vi "Write Test Configuration (INI) File_MultiTest.vi"(1 "# of Cycles(No \"T\")":string, 5 "ListBox_Selected_Tests":T1, 7 "FilePath in":path=path "C:/Users/DalLab/Desktop/Test Data", 10 "Filename: Date_LOT_Design_\"RCV\"":string, 11 "Experiments":T2={"Exp 1"={"Floor_Sweep_Stop_V"=36.0, "Resistance Threshold"=1000.0, "Floor_Sweep_Start_V"=0.0, "Floor_Sweep_Step_V"=1.0, "Roof_Sweep_Stop_V"=36.0, "Roof_Sweep_Start_V"=0.0, "Roof_Sweep_Step_V"=1.0, "Experiment Name"="", "Meas_Type"=[0, 2, 4]}, "Exp 2"={"Floor_Sweep_Stop_V"=36.0, "Resistance Threshold"=1000.0, "Floor_Sweep_Start_V"=0.0, "Floor_Sweep_Step_V"=1.0, "Roof_Sweep_Stop_V"=36.0, "Roof_Sweep_Start_V"=0.0, "Roof_Sweep_Step_V"=1.0, "Experiment Name"="", "Meas_Type"=[0, 2, 4]}, "Exp 3"={"Floor_Sweep_Stop_V"=36.0, "Resistance Threshold"=1000.0, "Floor_Sweep_Start_V"=0.0, "Floor_Sweep_Step_V"=1.0, "Roof_Sweep_Stop_V"=36.0, "Roof_Sweep_Start_V"=0.0, "Roof_Sweep_Step_V"=1.0, "Experiment Name"="", "Meas_Type"=[0, 2, 4]}, "Exp 4"={"Floor_Sweep_Stop_V"=36.0, "Resistance Threshold"=1000.0, "Floor_Sweep_Start_V"=0.0, "Floor_Sweep_Step_V"=1.0, "Roof_Sweep_Stop_V"=36.0, "Roof_Sweep_Start_V"=0.0, "Roof_Sweep_Step_V"=1.0, "Experiment Name"="", "Meas_Type"=[0, 2, 4]}}) -> (2 "Hold Down Time(Seconds) 2":dbl, 3 "Final Filepath Out":path)   [LabVIEW 2013]
doc: "Setup up to 4 different experiments. During SDR setup the specific experiments will be selected."
uses:
  Support/Controls/Multiple Exp Setup_MultiTest.ctl
  Support/Controls/Individual User Inputs_MultiTest.ctl
  Support/Controls/Test Selection.ctl
  <vilib>/Utility/config.llb/Write Key (String).vi
  <vilib>/Utility/config.llb/Write Key (Double).vi
  <vilib>/Utility/config.llb/Write Key (Path).vi
  <vilib>/Utility/config.llb/NI_LVConfig.lvlib
panel:
  in  "Hold Down Time(Seconds)":dbl=15.0
  in  "Save Button":bool
  # "Calculation Settings"
  # "Test Settings"
  # "Calculation Settings"
  # "Test Settings"
  # "Calculation Settings"
  # "Test Settings"
  # "Calculation Settings"
  # "Test Settings"
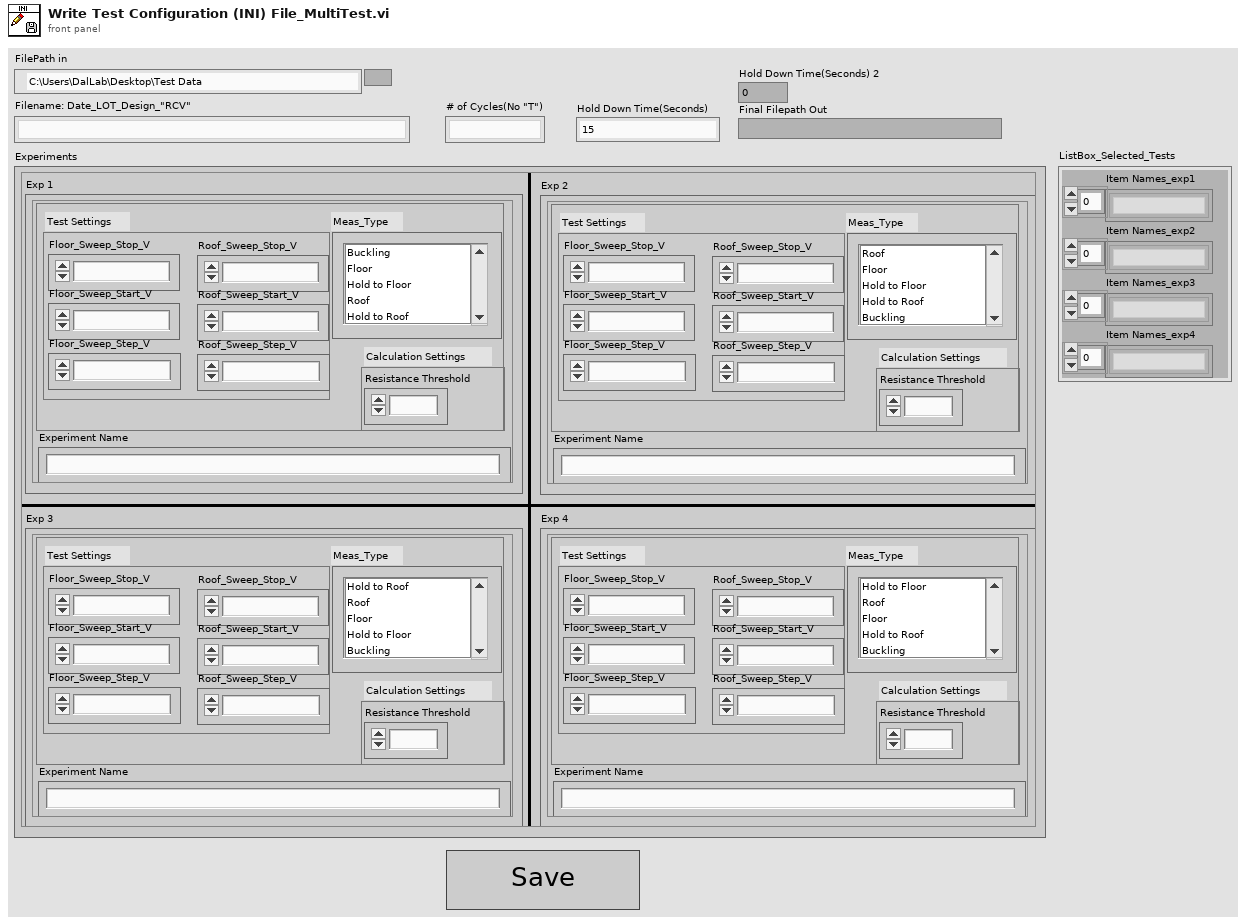
[diagram p1: front panel]
types:
  T1 = cluster{"Item Names_exp1":string[], "Item Names_exp2":string[], "Item Names_exp3":string[], "Item Names_exp4":string[]}
  T2 = typedef "Multiple Exp Setup_MultiTest.ctl" = cluster{"Exp 1":T3, "Exp 2":T3, "Exp 3":T3, "Exp 4":T3}
  T3 = typedef "Individual User Inputs_MultiTest.ctl" = cluster{"Floor_Sweep_Stop_V":dbl, "Resistance Threshold":dbl, "Floor_Sweep_Start_V":dbl, "Floor_Sweep_Step_V":dbl, "Roof_Sweep_Stop_V":dbl, "Roof_Sweep_Start_V":dbl, "Roof_Sweep_Step_V":dbl, "Experiment Name":string, "Meas_Type":T4}
  T4 = typedef "Test Selection.ctl" = i32[]
  T5 = typedef "NI_LVConfig.lvlib/Config Data RefNum.ctl" = refnum<k1>
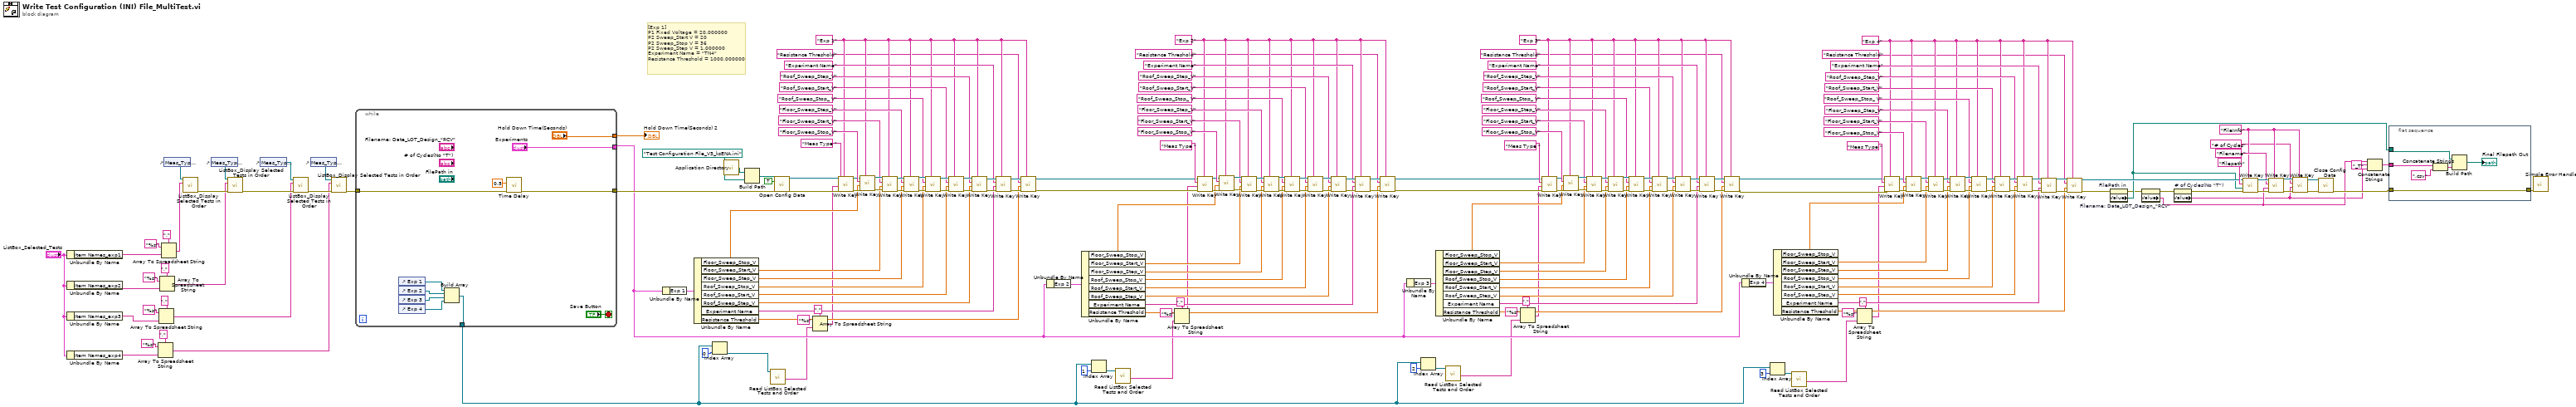
[diagram p0: block diagram]
diagram:
  w49 = "FileInfo" ("section")
  w114 = "Exp 4" ("section")
  w140 = "Exp 3" ("section")
  w166 = "Exp 2" ("section")
  w191 = "Exp 1" ("section")
  # "[Exp 1]\nP1 Fixed Voltage = 20.000000\nP2 Sweep_Start V = 20 \nP2 Sweep_Stop V = 36   \nP2 Sweep_Step V = 1.000000    \nExperiment Name = \"TN4\"\nResistance Threshold = 1000.000000"
  n1 = Unbundle By Name("ListBox_Selected_Tests") -> ("Item Names_exp1"=w22:string[])
  n2 = Unbundle By Name("ListBox_Selected_Tests") -> ("Item Names_exp2"=w9:string[])
  n3 = Unbundle By Name("ListBox_Selected_Tests") -> ("Item Names_exp3"=w6:string[])
  n4 = Unbundle By Name("ListBox_Selected_Tests") -> ("Item Names_exp4"=w7:string[])
  n5 = Array To Spreadsheet String(delimiter (Tab)=",", array=w7, 3:"%s" ("format string")) -> (spreadsheet string=w1:string)
  n6 = Array To Spreadsheet String(delimiter (Tab)=",", array=w6, 3:"%s" ("format string")) -> (spreadsheet string=w4:string)
  n7 = Array To Spreadsheet String(delimiter (Tab)=",", array=w9, 3:"%s" ("format string")) -> (spreadsheet string=w5:string)
  n8 = Array To Spreadsheet String(delimiter (Tab)=",", array=w22, 3:"%s" ("format string")) -> (spreadsheet string=w17:string)
  n9 = control-ref of="Meas_Type_Exp1"() -> (w18:refnum<vi>)
  n10 = call "ListBox_Display Selected Tests in Order.vi"("Tests"=w17, "Meas_Type_exp1"=w18) -> ("Error Out"=w19:errorcluster)  [unwired: 7 in, 2 out]
  n11 = control-ref of="Meas_Type_Exp2"() -> (w16:refnum<vi>)
  n12 = call "ListBox_Display Selected Tests in Order.vi"("Error In"=w19, "Tests"=w5, "Meas_Type_exp1"=w16) -> ("Error Out"=w20:errorcluster)  [unwired: 6 in, 2 out]
  n13 = control-ref of="Meas_Type_Exp3"() -> (w3:refnum<vi>)
  n14 = call "ListBox_Display Selected Tests in Order.vi"("Error In"=w20, "Tests"=w4, "Meas_Type_exp1"=w3) -> ("Error Out"=w21:errorcluster)  [unwired: 6 in, 2 out]
  n15 = control-ref of="Meas_Type_Exp4"() -> (w2:refnum<vi>)
  n16 = call "ListBox_Display Selected Tests in Order.vi"("Error In"=w21, "Tests"=w1, "Meas_Type_exp1"=w2) -> ("Error Out"=w25:errorcluster)  [unwired: 6 in, 2 out]
  n17 = while {
    tunnel: [w238] -> w219
    tunnel: ["Experiments"] -> w110
    tunnel: ["Hold Down Time(Seconds)"] -> w54
    tunnel: [w229] -> w37
    tunnel: w25 -> [w228]
    stop <- "Save Button" stop-if-true
    n18 = control-ref of="Exp 1"() -> (w233:refnum<vi>)
    n19 = control-ref of="Exp 2"() -> (w232:refnum<vi>)
    n20 = control-ref of="Exp 3"() -> (w231:refnum<vi>)
    n21 = control-ref of="Exp 4"() -> (w230:refnum<vi>)
    n22 = Build Array(w233, w232, w231, w230) -> (w229:refnum<vi>[])
    n23 = call "Time Delay"("error in (no error)"=w228, "Delay Time (s)"=0.5) -> ("error out"=w238:errorcluster)  [unwired: 9 in]
  }
  "Hold Down Time(Seconds) 2" <- w54
  n24 = Unbundle By Name(w110) -> ("Exp 1"=w210:T3)
  n25 = Unbundle By Name(w210) -> ("Floor_Sweep_Stop_V"=w208:dbl, "Floor_Sweep_Start_V"=w206:dbl, "Floor_Sweep_Step_V"=w204:dbl, "Roof_Sweep_Stop_V"=w202:dbl, "Roof_Sweep_Start_V"=w200:dbl, "Roof_Sweep_Step_V"=w198:dbl, "Experiment Name"=w192:string, "Resistance Threshold"=w189:dbl)
  n26 = Index Array(array=w37, index=0) -> (element=w26:refnum<vi>)
  n27 = call <vilib>:"Application Directory.vi"() -> ("Application Directory"=w222:path)
  n28 = Build Path(base path=w222, name or relative path=path "Test Configuration File_V3_ksENA.ini" ("default name")) -> (appended path=w223:path)
  n29 = call "Read ListBox Selected Tests and Order.vi"("Experiment Cluster"=w26) -> ("Per Exp Tests to Run"=w47:string[])  [unwired: 7 in, 3 out]
  n30 = call <vilib>:"Open Config Data.vi"("error in (no error)"=w219, "create file if necessary (T)"=TRUE ("create file if necessary? (T)"), "configuration file path"=w223) -> ("error out"=w70:errorcluster, "refnum"=w84:T5)  [unwired: 6 in, 1 out]
  n31 = Array To Spreadsheet String(delimiter (Tab)=",", array=w47, 3:"%s" ("format string")) -> (spreadsheet string=w69:string)
  n32 = call-poly <vilib>:"Write Key.vi"("section"=w191, "error in (no error)"=w70, "value"=w69, "key"="Meas Type " ("Key 1"), "refnum"=w84) -> ("error out"=w212:errorcluster, "refnum out"=w83:T5)  [unwired: 4 in, 1 out]
  n33 = call-poly <vilib>:"Write Key.vi"("section"=w191, "error in (no error)"=w212, "value"=w208, "key"="Floor_Sweep_Stop_V" ("Key 2"), "refnum"=w83) -> ("error out"=w218:errorcluster, "refnum out"=w217:T5)  [unwired: 4 in, 1 out]
  n34 = call-poly <vilib>:"Write Key.vi"("section"=w191, "error in (no error)"=w218, "value"=w206, "key"="Floor_Sweep_Start_V" ("Key 2"), "refnum"=w217) -> ("error out"=w215:errorcluster, "refnum out"=w216:T5)  [unwired: 4 in, 1 out]
  n35 = call-poly <vilib>:"Write Key.vi"("section"=w191, "error in (no error)"=w215, "value"=w204, "key"="Floor_Sweep_Step_V" ("Key 2"), "refnum"=w216) -> ("error out"=w224:errorcluster, "refnum out"=w225:T5)  [unwired: 4 in, 1 out]
  n36 = call-poly <vilib>:"Write Key.vi"("section"=w191, "error in (no error)"=w224, "value"=w202, "key"="Roof_Sweep_Stop_ V" ("Key 3"), "refnum"=w225) -> ("error out"=w221:errorcluster, "refnum out"=w220:T5)  [unwired: 4 in, 1 out]
  n37 = call-poly <vilib>:"Write Key.vi"("section"=w191, "error in (no error)"=w221, "value"=w200, "key"="Roof_Sweep_Start_V" ("Key 3"), "refnum"=w220) -> ("error out"=w214:errorcluster, "refnum out"=w213:T5)  [unwired: 4 in, 1 out]
  n38 = call-poly <vilib>:"Write Key.vi"("section"=w191, "error in (no error)"=w214, "value"=w198, "key"="Roof_Sweep_Step_V" ("Key 3"), "refnum"=w213) -> ("error out"=w196:errorcluster, "refnum out"=w195:T5)  [unwired: 4 in, 1 out]
  n39 = call-poly <vilib>:"Write Key.vi"("section"=w191, "error in (no error)"=w196, "value"=w192, "key"="Experiment Name" ("Key 3"), "refnum"=w195) -> ("error out"=w197:errorcluster, "refnum out"=w194:T5)  [unwired: 4 in, 1 out]
  n40 = call-poly <vilib>:"Write Key.vi"("section"=w191, "error in (no error)"=w197, "value"=w189, "key"="Resistance Threshold" ("Key 3"), "refnum"=w194) -> ("error out"=w63:errorcluster, "refnum out"=w82:T5)  [unwired: 4 in, 1 out]
  n41 = Unbundle By Name(w110) -> ("Exp 2"=w164:T3)
  n42 = Unbundle By Name(w164) -> ("Floor_Sweep_Stop_V"=w109:dbl, "Floor_Sweep_Start_V"=w108:dbl, "Floor_Sweep_Step_V"=w107:dbl, "Roof_Sweep_Stop_V"=w106:dbl, "Roof_Sweep_Start_V"=w105:dbl, "Roof_Sweep_Step_V"=w104:dbl, "Experiment Name"=w103:string, "Resistance Threshold"=w102:dbl)
  n43 = Index Array(array=w37, index=1) -> (element=w41:refnum<vi>)
  n44 = call "Read ListBox Selected Tests and Order.vi"("Experiment Cluster"=w41) -> ("Per Exp Tests to Run"=w46:string[])  [unwired: 7 in, 3 out]
  n45 = Array To Spreadsheet String(delimiter (Tab)=",", array=w46, 3:"%s" ("format string")) -> (spreadsheet string=w61:string)
  n46 = call-poly <vilib>:"Write Key.vi"("section"=w166, "error in (no error)"=w63, "value"=w61, "key"="Meas Type " ("Key 1"), "refnum"=w82) -> ("error out"=w178:errorcluster, "refnum out"=w81:T5)  [unwired: 4 in, 1 out]
  n47 = call-poly <vilib>:"Write Key.vi"("section"=w166, "error in (no error)"=w178, "value"=w109, "key"="Floor_Sweep_Stop_V" ("Key 2"), "refnum"=w81) -> ("error out"=w184:errorcluster, "refnum out"=w183:T5)  [unwired: 4 in, 1 out]
  n48 = call-poly <vilib>:"Write Key.vi"("section"=w166, "error in (no error)"=w184, "value"=w108, "key"="Floor_Sweep_Start_V" ("Key 2"), "refnum"=w183) -> ("error out"=w181:errorcluster, "refnum out"=w182:T5)  [unwired: 4 in, 1 out]
  n49 = call-poly <vilib>:"Write Key.vi"("section"=w166, "error in (no error)"=w181, "value"=w107, "key"="Floor_Sweep_Step_V" ("Key 2"), "refnum"=w182) -> ("error out"=w187:errorcluster, "refnum out"=w188:T5)  [unwired: 4 in, 1 out]
  n50 = call-poly <vilib>:"Write Key.vi"("section"=w166, "error in (no error)"=w187, "value"=w106, "key"="Roof_Sweep_Stop_ V" ("Key 3"), "refnum"=w188) -> ("error out"=w186:errorcluster, "refnum out"=w185:T5)  [unwired: 4 in, 1 out]
  n51 = call-poly <vilib>:"Write Key.vi"("section"=w166, "error in (no error)"=w186, "value"=w105, "key"="Roof_Sweep_Start_V" ("Key 3"), "refnum"=w185) -> ("error out"=w180:errorcluster, "refnum out"=w179:T5)  [unwired: 4 in, 1 out]
  n52 = call-poly <vilib>:"Write Key.vi"("section"=w166, "error in (no error)"=w180, "value"=w104, "key"="Roof_Sweep_Step_V" ("Key 3"), "refnum"=w179) -> ("error out"=w170:errorcluster, "refnum out"=w169:T5)  [unwired: 4 in, 1 out]
  n53 = call-poly <vilib>:"Write Key.vi"("section"=w166, "error in (no error)"=w170, "value"=w103, "key"="Experiment Name" ("Key 3"), "refnum"=w169) -> ("error out"=w171:errorcluster, "refnum out"=w168:T5)  [unwired: 4 in, 1 out]
  n54 = call-poly <vilib>:"Write Key.vi"("section"=w166, "error in (no error)"=w171, "value"=w102, "key"="Resistance Threshold" ("Key 3"), "refnum"=w168) -> ("error out"=w60:errorcluster, "refnum out"=w80:T5)  [unwired: 4 in, 1 out]
  n55 = Unbundle By Name(w110) -> ("Exp 3"=w137:T3)
  n56 = Index Array(array=w37, index=2) -> (element=w39:refnum<vi>)
  n57 = Unbundle By Name(w137) -> ("Floor_Sweep_Stop_V"=w101:dbl, "Floor_Sweep_Start_V"=w100:dbl, "Floor_Sweep_Step_V"=w99:dbl, "Roof_Sweep_Stop_V"=w98:dbl, "Roof_Sweep_Start_V"=w97:dbl, "Roof_Sweep_Step_V"=w96:dbl, "Experiment Name"=w95:string, "Resistance Threshold"=w94:dbl)
  n58 = call "Read ListBox Selected Tests and Order.vi"("Experiment Cluster"=w39) -> ("Per Exp Tests to Run"=w45:string[])  [unwired: 7 in, 3 out]
  n59 = Array To Spreadsheet String(delimiter (Tab)=",", array=w45, 3:"%s" ("format string")) -> (spreadsheet string=w58:string)
  n60 = call-poly <vilib>:"Write Key.vi"("section"=w140, "error in (no error)"=w60, "value"=w58, "key"="Meas Type " ("Key 1"), "refnum"=w80) -> ("error out"=w152:errorcluster, "refnum out"=w85:T5)  [unwired: 4 in, 1 out]
  n61 = call-poly <vilib>:"Write Key.vi"("section"=w140, "error in (no error)"=w152, "value"=w101, "key"="Floor_Sweep_Stop_V" ("Key 2"), "refnum"=w85) -> ("error out"=w158:errorcluster, "refnum out"=w157:T5)  [unwired: 4 in, 1 out]
  n62 = call-poly <vilib>:"Write Key.vi"("section"=w140, "error in (no error)"=w158, "value"=w100, "key"="Floor_Sweep_Start_V" ("Key 2"), "refnum"=w157) -> ("error out"=w155:errorcluster, "refnum out"=w156:T5)  [unwired: 4 in, 1 out]
  n63 = call-poly <vilib>:"Write Key.vi"("section"=w140, "error in (no error)"=w155, "value"=w99, "key"="Floor_Sweep_Step_V" ("Key 2"), "refnum"=w156) -> ("error out"=w161:errorcluster, "refnum out"=w162:T5)  [unwired: 4 in, 1 out]
  n64 = call-poly <vilib>:"Write Key.vi"("section"=w140, "error in (no error)"=w161, "value"=w98, "key"="Roof_Sweep_Stop_ V" ("Key 3"), "refnum"=w162) -> ("error out"=w160:errorcluster, "refnum out"=w159:T5)  [unwired: 4 in, 1 out]
  n65 = call-poly <vilib>:"Write Key.vi"("section"=w140, "error in (no error)"=w160, "value"=w97, "key"="Roof_Sweep_Start_V" ("Key 3"), "refnum"=w159) -> ("error out"=w154:errorcluster, "refnum out"=w153:T5)  [unwired: 4 in, 1 out]
  n66 = call-poly <vilib>:"Write Key.vi"("section"=w140, "error in (no error)"=w154, "value"=w96, "key"="Roof_Sweep_Step_V" ("Key 3"), "refnum"=w153) -> ("error out"=w144:errorcluster, "refnum out"=w143:T5)  [unwired: 4 in, 1 out]
  n67 = call-poly <vilib>:"Write Key.vi"("section"=w140, "error in (no error)"=w144, "value"=w95, "key"="Experiment Name" ("Key 3"), "refnum"=w143) -> ("error out"=w145:errorcluster, "refnum out"=w142:T5)  [unwired: 4 in, 1 out]
  n68 = call-poly <vilib>:"Write Key.vi"("section"=w140, "error in (no error)"=w145, "value"=w94, "key"="Resistance Threshold" ("Key 3"), "refnum"=w142) -> ("error out"=w57:errorcluster, "refnum out"=w79:T5)  [unwired: 4 in, 1 out]
  n69 = Unbundle By Name(w110) -> ("Exp 4"=w111:T3)
  n70 = Index Array(array=w37, index=3) -> (element=w36:refnum<vi>)
  n71 = Unbundle By Name(w111) -> ("Floor_Sweep_Stop_V"=w93:dbl, "Floor_Sweep_Start_V"=w92:dbl, "Floor_Sweep_Step_V"=w91:dbl, "Roof_Sweep_Stop_V"=w90:dbl, "Roof_Sweep_Start_V"=w89:dbl, "Roof_Sweep_Step_V"=w88:dbl, "Experiment Name"=w87:string, "Resistance Threshold"=w86:dbl)
  n72 = call "Read ListBox Selected Tests and Order.vi"("Experiment Cluster"=w36) -> ("Per Exp Tests to Run"=w44:string[])  [unwired: 7 in, 3 out]
  n73 = Array To Spreadsheet String(delimiter (Tab)=",", array=w44, 3:"%s" ("format string")) -> (spreadsheet string=w55:string)
  n74 = call-poly <vilib>:"Write Key.vi"("section"=w114, "error in (no error)"=w57, "value"=w55, "key"="Meas Type " ("Key 1"), "refnum"=w79) -> ("error out"=w126:errorcluster, "refnum out"=w78:T5)  [unwired: 4 in, 1 out]
  n75 = call-poly <vilib>:"Write Key.vi"("section"=w114, "error in (no error)"=w126, "value"=w93, "key"="Floor_Sweep_Stop_V" ("Key 2"), "refnum"=w78) -> ("error out"=w132:errorcluster, "refnum out"=w131:T5)  [unwired: 4 in, 1 out]
  n76 = call-poly <vilib>:"Write Key.vi"("section"=w114, "error in (no error)"=w132, "value"=w92, "key"="Floor_Sweep_Start_V" ("Key 2"), "refnum"=w131) -> ("error out"=w129:errorcluster, "refnum out"=w130:T5)  [unwired: 4 in, 1 out]
  n77 = call-poly <vilib>:"Write Key.vi"("section"=w114, "error in (no error)"=w129, "value"=w91, "key"="Floor_Sweep_Step_V" ("Key 2"), "refnum"=w130) -> ("error out"=w135:errorcluster, "refnum out"=w136:T5)  [unwired: 4 in, 1 out]
  n78 = call-poly <vilib>:"Write Key.vi"("section"=w114, "error in (no error)"=w135, "value"=w90, "key"="Roof_Sweep_Stop_ V" ("Key 3"), "refnum"=w136) -> ("error out"=w134:errorcluster, "refnum out"=w133:T5)  [unwired: 4 in, 1 out]
  n79 = call-poly <vilib>:"Write Key.vi"("section"=w114, "error in (no error)"=w134, "value"=w89, "key"="Roof_Sweep_Start_V" ("Key 3"), "refnum"=w133) -> ("error out"=w128:errorcluster, "refnum out"=w127:T5)  [unwired: 4 in, 1 out]
  n80 = call-poly <vilib>:"Write Key.vi"("section"=w114, "error in (no error)"=w128, "value"=w88, "key"="Roof_Sweep_Step_V" ("Key 3"), "refnum"=w127) -> ("error out"=w118:errorcluster, "refnum out"=w117:T5)  [unwired: 4 in, 1 out]
  n81 = call-poly <vilib>:"Write Key.vi"("section"=w114, "error in (no error)"=w118, "value"=w87, "key"="Experiment Name" ("Key 3"), "refnum"=w117) -> ("error out"=w119:errorcluster, "refnum out"=w116:T5)  [unwired: 4 in, 1 out]
  n82 = call-poly <vilib>:"Write Key.vi"("section"=w114, "error in (no error)"=w119, "value"=w86, "key"="Resistance Threshold" ("Key 3"), "refnum"=w116) -> ("error out"=w33:errorcluster, "refnum out"=w71:T5)  [unwired: 4 in, 1 out]
  n83 = property on="FilePath in" class="Path"(error in=w33) -> (error out=w34:errorcluster, "Value"=w35:path)  [unwired: 1 in, 1 out]
  n84 = property on="Filename: Date_LOT_Design_\"RCV\"" class="Str"(error in=w34) -> (error out=w32:errorcluster, "Value"=w28:string)  [unwired: 1 in, 1 out]
  n85 = property on="# of Cycles(No \"T\")" class="Str"(error in=w32) -> (error out=w31:errorcluster, "Value"=w27:string)  [unwired: 1 in, 1 out]
  n86 = call-poly <vilib>:"Write Key.vi"("section"=w49, "error in (no error)"=w31, "value"=w35, "key"="Filepath" ("Key 1"), "refnum"=w71) -> ("error out"=w75:errorcluster, "refnum out"=w74:T5)  [unwired: 4 in, 1 out]
  n87 = call-poly <vilib>:"Write Key.vi"("section"=w49, "error in (no error)"=w75, "value"=w28, "key"="Filename" ("Key 1"), "refnum"=w74) -> ("error out"=w53:errorcluster, "refnum out"=w50:T5)  [unwired: 4 in, 1 out]
  n88 = call-poly <vilib>:"Write Key.vi"("section"=w49, "error in (no error)"=w53, "value"=w27, "key"="# of Cycles" ("Key 1"), "refnum"=w50) -> ("error out"=w52:errorcluster, "refnum out"=w51:T5)  [unwired: 4 in, 1 out]
  n89 = call <vilib>:"Close Config Data.vi"("error in (no error)"=w52, "refnum"=w51) -> ("error out"=w77:errorcluster)  [unwired: 1 in, 8 out]
  n90 = Concatenate Strings(w28, "_T", w27) -> (w29:string)
  n91 = flat-sequence {
    tunnel: w77 -> [w243]
    tunnel: [w243] -> w76
    tunnel: w35 -> [w242]
    tunnel: w29 -> [w239]
    frame #0 {
      n92 = Concatenate Strings(w239, ".csv" ("string")) -> (w241:string)
      n93 = Build Path(base path=w242, name or relative path=w241) -> (appended path=→"Final Filepath Out":path)
    }
  }
  n94 = call <vilib>:"Simple Error Handler.vi"("error in (no error)"=w76) -> ()  [unwired: 2 in, 7 out]
